vi "Init.vi"(5 "Instrument.lvclass 2":refnum<class "Instrument.lvclass">, 6 "Step":dbl, 7 "Instrument.lvclass":refnum<class "Instrument.lvclass">, 8 "error in (no error)":errorcluster, 9 "Max":dbl, 10 "Init":dbl, 11 "Measurement1D in":refnum<class "IV_meas.lvclass">) -> (0 "error out":errorcluster, 3 "Measurement1D out":refnum<class "IV_meas.lvclass">)   [LabVIEW 2018, in "IV_meas.lvclass"]
uses:
  IV_meas.lvclass
  Abstract/Instrument/Instrument/Instrument.lvclass
  Abstract/Measurement/Measurement2D/Measurement2D.lvclass
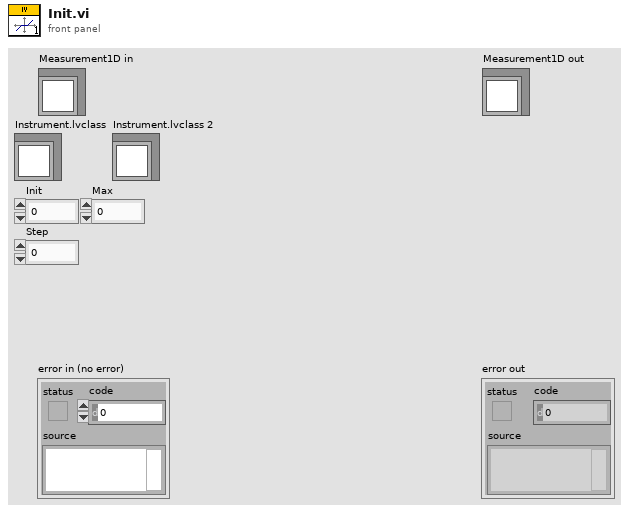
[diagram p1: front panel]
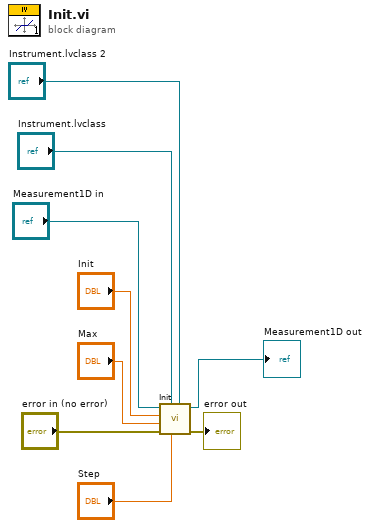
[diagram p0: block diagram]
diagram:
  n1 = call-parent "Init.vi"("Instrument.lvclass 2"="Instrument.lvclass 2", "Step"="Step", "Instrument 1.lvclass"="Instrument.lvclass", "error in (no error)"="error in (no error)", "Max"="Max", "Init"="Init", "Measurement1D in"="Measurement1D in") -> ("error out"=→"error out":errorcluster, "Measurement1D out"=→"Measurement1D out":refnum<class "IV_meas.lvclass">)  [unwired: 3 in]
